vi "Determine Warnings.vi"(8 "Error In":errorcluster) -> (0 "Error Out":errorcluster)   [LabVIEW 2020]
panel:
  in  "Warning Text":string
  in  "Warning?":bool
  in  "Min Temperature":dbl
  in  "Max Temperature":dbl
  in  "Current Temperature":dbl
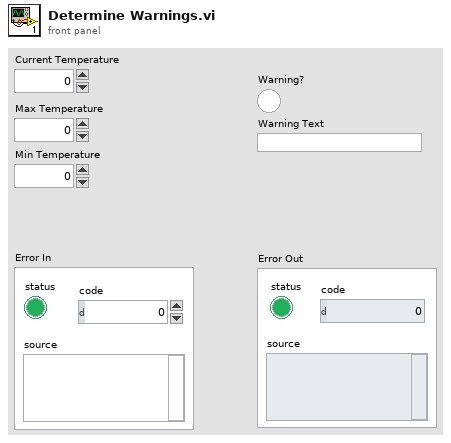
[diagram p1: front panel]
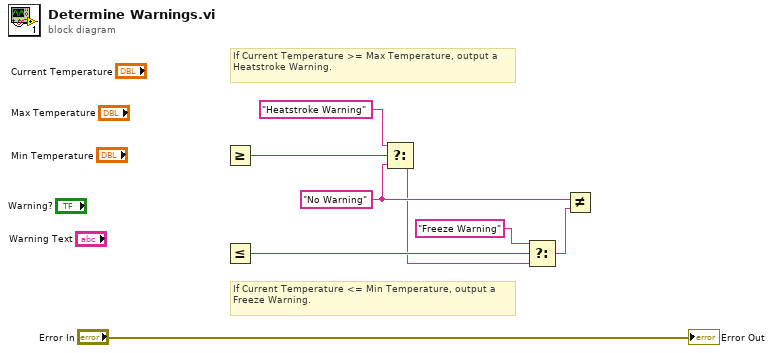
[diagram p0: block diagram]
diagram:
  w5 = "No Warning"
  # "If Current Temperature <= Min Temperature, output a Freeze Warning."
  # "If Current Temperature >= Max Temperature, output a Heatstroke Warning."
  n1 = Greater Or Equal?() -> (x >= y?=w8:bool)  [unwired: 2 in]
  n2 = Less Or Equal?() -> (x <= y?=w6:bool)  [unwired: 2 in]
  n3 = Select(t="Heatstroke Warning", s=w8, f=w5) -> (s? t:f=w4:string)
  n4 = Select(t="Freeze Warning", s=w6, f=w4) -> (s? t:f=w1:string)
  n5 = Not Equal?(x=w5, y=w1) -> ()  [unwired: 1 out]
  "Error Out" <- "Error In"
